vi "Scaled XOR Data.vi"() -> (6 "XOR File Out":path, 8 "XOR_VAL File Out":path)   [LabVIEW 2015]
uses:
  Teaching File/Teaching File.lvlib
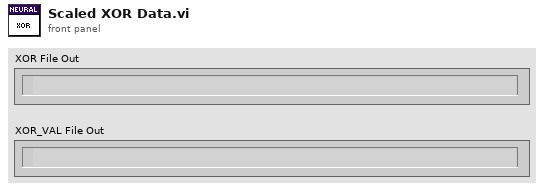
[diagram p1: front panel]
types:
  T1 = enum16{"open", "open or create", "create or replace", "create", "open (read-only)"}
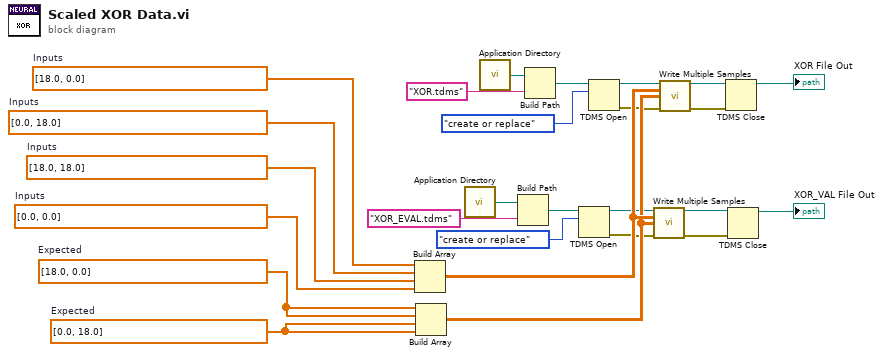
[diagram p0: block diagram]
diagram:
  w15 = dbl[] [0.0, 18.0]  # Expected
  w17 = dbl[] [0.0, 0.0]  # Inputs
  w18 = dbl[] [18.0, 18.0]  # Inputs
  w19 = dbl[] [0.0, 18.0]  # Inputs
  w16 = dbl[] [18.0, 0.0]  # Expected
  w20 = dbl[] [18.0, 0.0]  # Inputs
  n1 = Build Array(w20, w19, w18, w17) -> (w14:dbl[][])
  n2 = Build Array(w16, w16, w15, w15) -> (w13:dbl[][])
  n3 = call <vilib>:"Application Directory.vi"() -> ("Application Directory"=w22:path)
  n4 = call <vilib>:"Application Directory.vi"() -> ("Application Directory"=w26:path)
  n5 = Build Path(base path=w22, name or relative path="XOR_EVAL.tdms") -> (appended path=w6:path)
  n6 = Build Path(base path=w26, name or relative path="XOR.tdms") -> (appended path=w3:path)
  n7 = TDMS Open(10:T1."create or replace" ("operation (0:open)"), 11:w6) -> (0:w7:errorcluster, 3:w8:refnum<k34>)  [unwired: 5 in]
  n8 = TDMS Open(10:T1."create or replace" ("operation (0:open)"), 11:w3) -> (0:w1:errorcluster, 3:w2:refnum<k34>)  [unwired: 5 in]
  n9 = call "Write Multiple Samples.vi"("TDMS In"=w8, "Input Vector"=w14, "Output Vector"=w13, "Error In"=w7) -> ("TDMS Out"=w21:refnum<k34>, "Error Out"=w12:errorcluster)  [unwired: 10 in]
  n10 = call "Write Multiple Samples.vi"("TDMS In"=w2, "Input Vector"=w14, "Output Vector"=w13, "Error In"=w1) -> ("TDMS Out"=w11:refnum<k34>, "Error Out"=w10:errorcluster)  [unwired: 10 in]
  n11 = TDMS Close(8:w10, 11:w11) -> (3:→"XOR File Out":path)  [unwired: 1 out]
  n12 = TDMS Close(8:w12, 11:w21) -> (3:→"XOR_VAL File Out":path)  [unwired: 1 out]
